vi "Do.vi"(8 "error in (no error)":errorcluster, 10 "Parent Actor":refnum<class "Parent Actor.lvclass">, 11 "Parent Message in":refnum<class "Parent Message.lvclass">) -> (0 "error out":errorcluster, 2 "Parent Actor out":refnum<class "Parent Actor.lvclass">, 3 "Parent Message out":refnum<class "Parent Message.lvclass">)   [LabVIEW 2015, in "Parent Message.lvclass"]
uses:
  Parent Message.lvclass
  State/Parent Actor.lvclass
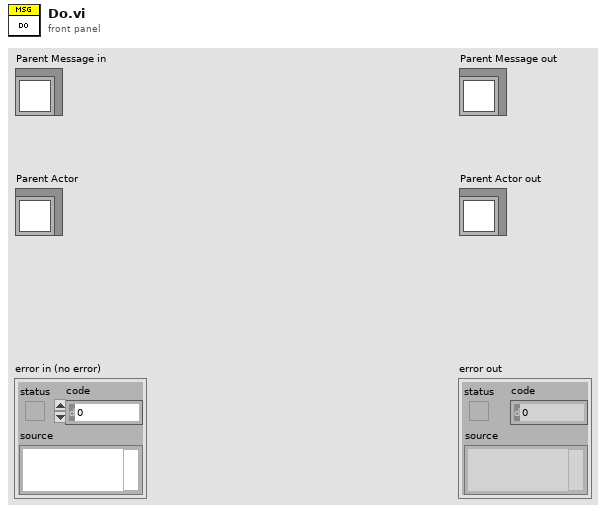
[diagram p1: front panel]
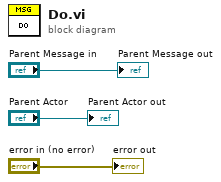
[diagram p0: block diagram]
diagram:
  "error out" <- "error in (no error)"
  "Parent Message out" <- "Parent Message in"
  "Parent Actor out" <- "Parent Actor"
